vi "piezo.vi"() -> ()   [LabVIEW 2017]
uses:
  C:/Users/Li Lab/Documents/LabVIEW Data/kinesis_test - 3/Thorlabs.MotionControl.Controls.dll
  Thorlabs.MotionControl.Controls.dll
  System.Windows.Forms
  C:/Users/Li Lab/Documents/LabVIEW Data/kinesis_test - 3/Thorlabs.MotionControl.KCube.InertialMotorCLI.dll
  Thorlabs.MotionControl.KCube.InertialMotorCLI.dll
  C:/Users/Li Lab/Documents/LabVIEW Data/kinesis_test - 3/ThorLabs.MotionControl.KCube.DCServoCLI.dll
  ThorLabs.MotionControl.KCube.DCServoCLI.dll
  C:/Program Files/Thorlabs/Scientific Imaging/DCx Camera Support/Develop/DotNet/uc480DotNet.dll
  Program Files/Thorlabs/Scientific Imaging/DCx Camera Support/Develop/DotNet/uc480DotNet.dll
  <vilib>/Utility/inputDevices.llb/mouseAcquire.vi
  <vilib>/Utility/inputDevices.llb/joystickAcquire.vi
  <vilib>/Utility/inputDevices.llb/closeMouse.vi
  <vilib>/Utility/inputDevices.llb/closeJoystick.vi
panel:
  out "blinker and move":bool
  out "in screen?":bool
  in  "ready to use mouse?":bool
  out "Numeric1":dbl
  out "Numeric2":dbl
  out "motor 1":dbl
  out "motor 2":dbl
  out "Moving":bool
  in  "1mm=?pixel":i32
  in  "Motor Display":T1(tab)
  in  "KCubeInertialMotorControl":refnum<k24>(container)
  in  "KCubeDCServoControl-motor 1":refnum<k24>(container)
  in  "KCubeDCServoControl-motor 2":refnum<k24>(container)
  out "error out 9":errorcluster
  out "error out 8":errorcluster
  in  "PictureBox":refnum<k24>(container)
  in  "Init Camera":bool
  in  "Start Live":bool
  in  "Exit Camera":bool
  in  "Stop Live":bool
  in  "Load Parameter":bool
  out "Error Out":errorcluster caption="error"
  out "Bits/Pixel 2":i32=8
  out "Width 2":i32=8
  out "Height 2":i32=8
  out "Serial Number 2":string
  out "Position of z direction":i32
  in  "?":bool
  in  "Input Box":T2(tab)
  in  "a":dbl
  in  "b":dbl
  in  "c":dbl
  in  "d":dbl
  out "upper verti limit":dbl
  out "lower verti limit":dbl
  out "left hori limit":dbl
  out "right hori limit":dbl
  out "Horizontal":i32
  out "Vertical":i32
  out "Scrolling":i32
  out "button 1":bool
  out "button 2":bool
  out "Horizontal right click":i32
  out "Vertical right click":i32
  out "Horizontal left click":i32
  out "Vertical left click":i32
  in  "Pixelclock":i32(slide)=33 min=5 max=43 step=1 scale=5.0..43.0
  in  "Framerate":dbl(slide)=33.21525 min=4.876716604244694 max=13.962044182888818 step=0.013000041138630184 scale=4.876716604244694..13.962044182888818 scale format="%#.3g"
  in  "Exposure":dbl(slide)=33.21525 min=0.06675 max=99.92475 step=0.06675 scale=0.06675..99.92475 scale format="%#.3g"
  in  "Zoom":u16(ring)=1 items=["4X"=4, "2X"=2, "1X"=1]
  in  "Camera ID":i32
  out "Serial Number":string
  out "Height":i32=8
  out "Width":i32=8
  out "Bits/Pixel":i32=8
  in  "SerialNumber KDC101 2":string="27251775"
  in  "SerialNumber KDC101":string="27251750"
  in  "SerialNumber  of KIM101":string="97000019"
  out "Time the program is running (s)":dbl caption="Elapsed Time (s)"
  out "You are Sprinting now":bool
  in  "channel 3":i32(ring)=1 items=["Channel1"=1, "Channel2"=2, "Channel3"=3, "Channel4"=4]
  in  "stop 2":bool
  in  "stop":bool
  in  "Cancel Button":bool
  in  "Move motor control":bool
  in  "step size (mm) 2":dbl
  in  "end pos (mm)":dbl
  out "Move motor indicator":bool
  out "position of motor 2 (mm)":dbl
  out "error out 7":errorcluster
  out "error out 6":errorcluster
  out "error out 4":errorcluster
  out "error out 3":errorcluster
  out "error out 2":errorcluster
  out "error out":errorcluster
  out "error out 5":errorcluster
  out "position of motor 1 (mm)":dbl
  out "direction info 2":T3
  out "axis info 2":T4
  out "button info 2":T5
  # "left is off, right is on"
  # "Li Lab, Camera and Microscope Stage Controller"
  # "1. Right Click on the laser point and left click where you want to move it\n2. Please Exit camera before closing the program, please, please, please!!!!!\n3. Enter the mm to pixel convertion before moving the mouse.\n4. All the input controls can be found on the Input Control Box!\n5. If any Bugs found please contact deyraunak111@gmail.com\n6. A video or photo recording version will come up shortly, until that use the Thorlabs camera.\n7. Set the laser position and the screen before trying to capture the bead with the mouse. Look at the convention and input the \nvalues of a,b,c,d. Then turn the knob to use mouse. Enjoy!"
  # "laser pointer"
  # "Axis convention:"
  # "up is negative down is positiive, right is positive left is negative"
  # "This feature is non functional now for the time being"
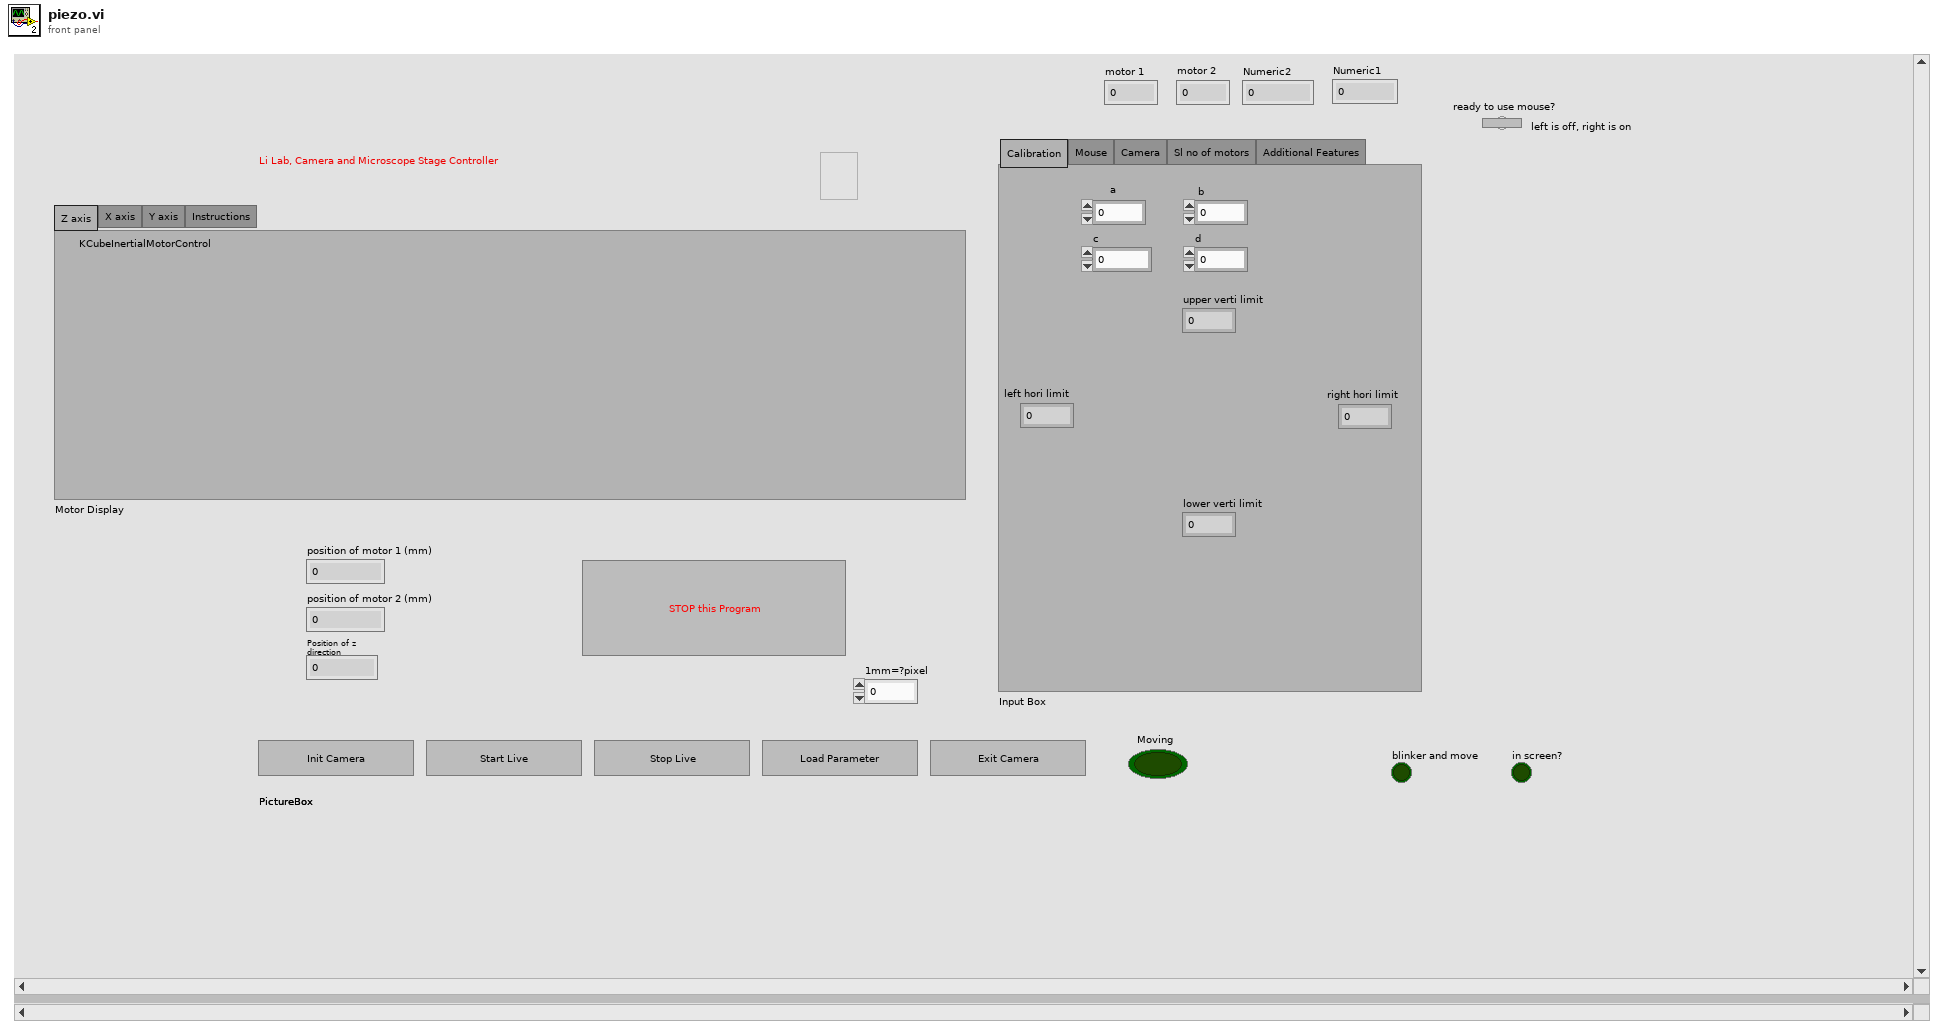
[diagram p1: front panel]
types:
  T1 = enum32{"Z axis", "X axis", "Y axis", "Instructions"}
  T2 = enum32{"Calibration", "Mouse", "Camera", "Sl no of motors", "Additional Features"}
  T3 = cluster{"pov 1":i32, "pov 2":i32, "pov 3":i32, "pov 4":i32}
  T4 = cluster{"X axis":i32, "Y axis":i32, "Z axis":i32, "X axis rotation":i32, "Y axis rotation":i32, "Z axis rotation":i32, "U axis":i32, "V axis":i32}
  T5 = cluster{"button 1":bool, "button 2":bool, "button 3":bool, "button 4":bool, "button 5":bool, "button 6":bool, "button 7":bool, "button 8":bool, "button 9":bool, "button 10":bool, "button 11":bool, "button 12":bool, "button 13":bool, "button 14":bool, "button 15":bool, "button 16":bool, "button 17":bool, "button 18":bool, "button 19":bool, "button 20":bool, "button 21":bool, "button 22":bool, "button 23":bool, "button 24":bool, "button 25":bool, "button 26":bool, "button 27":bool, "button 28":bool, "button 29":bool, "button 30":bool, "button 31":bool, "button 32":bool}
  T6 = enum8{"Enabled", "Disabled", "Disabled and Grayed Out"}
  T7 = cluster{"Horizontal":i32, "Vertical":i32, "Scrolling":i32}
  T8 = cluster{"button 1":bool, "button 2":bool, "button 3":bool, "button 4":bool}
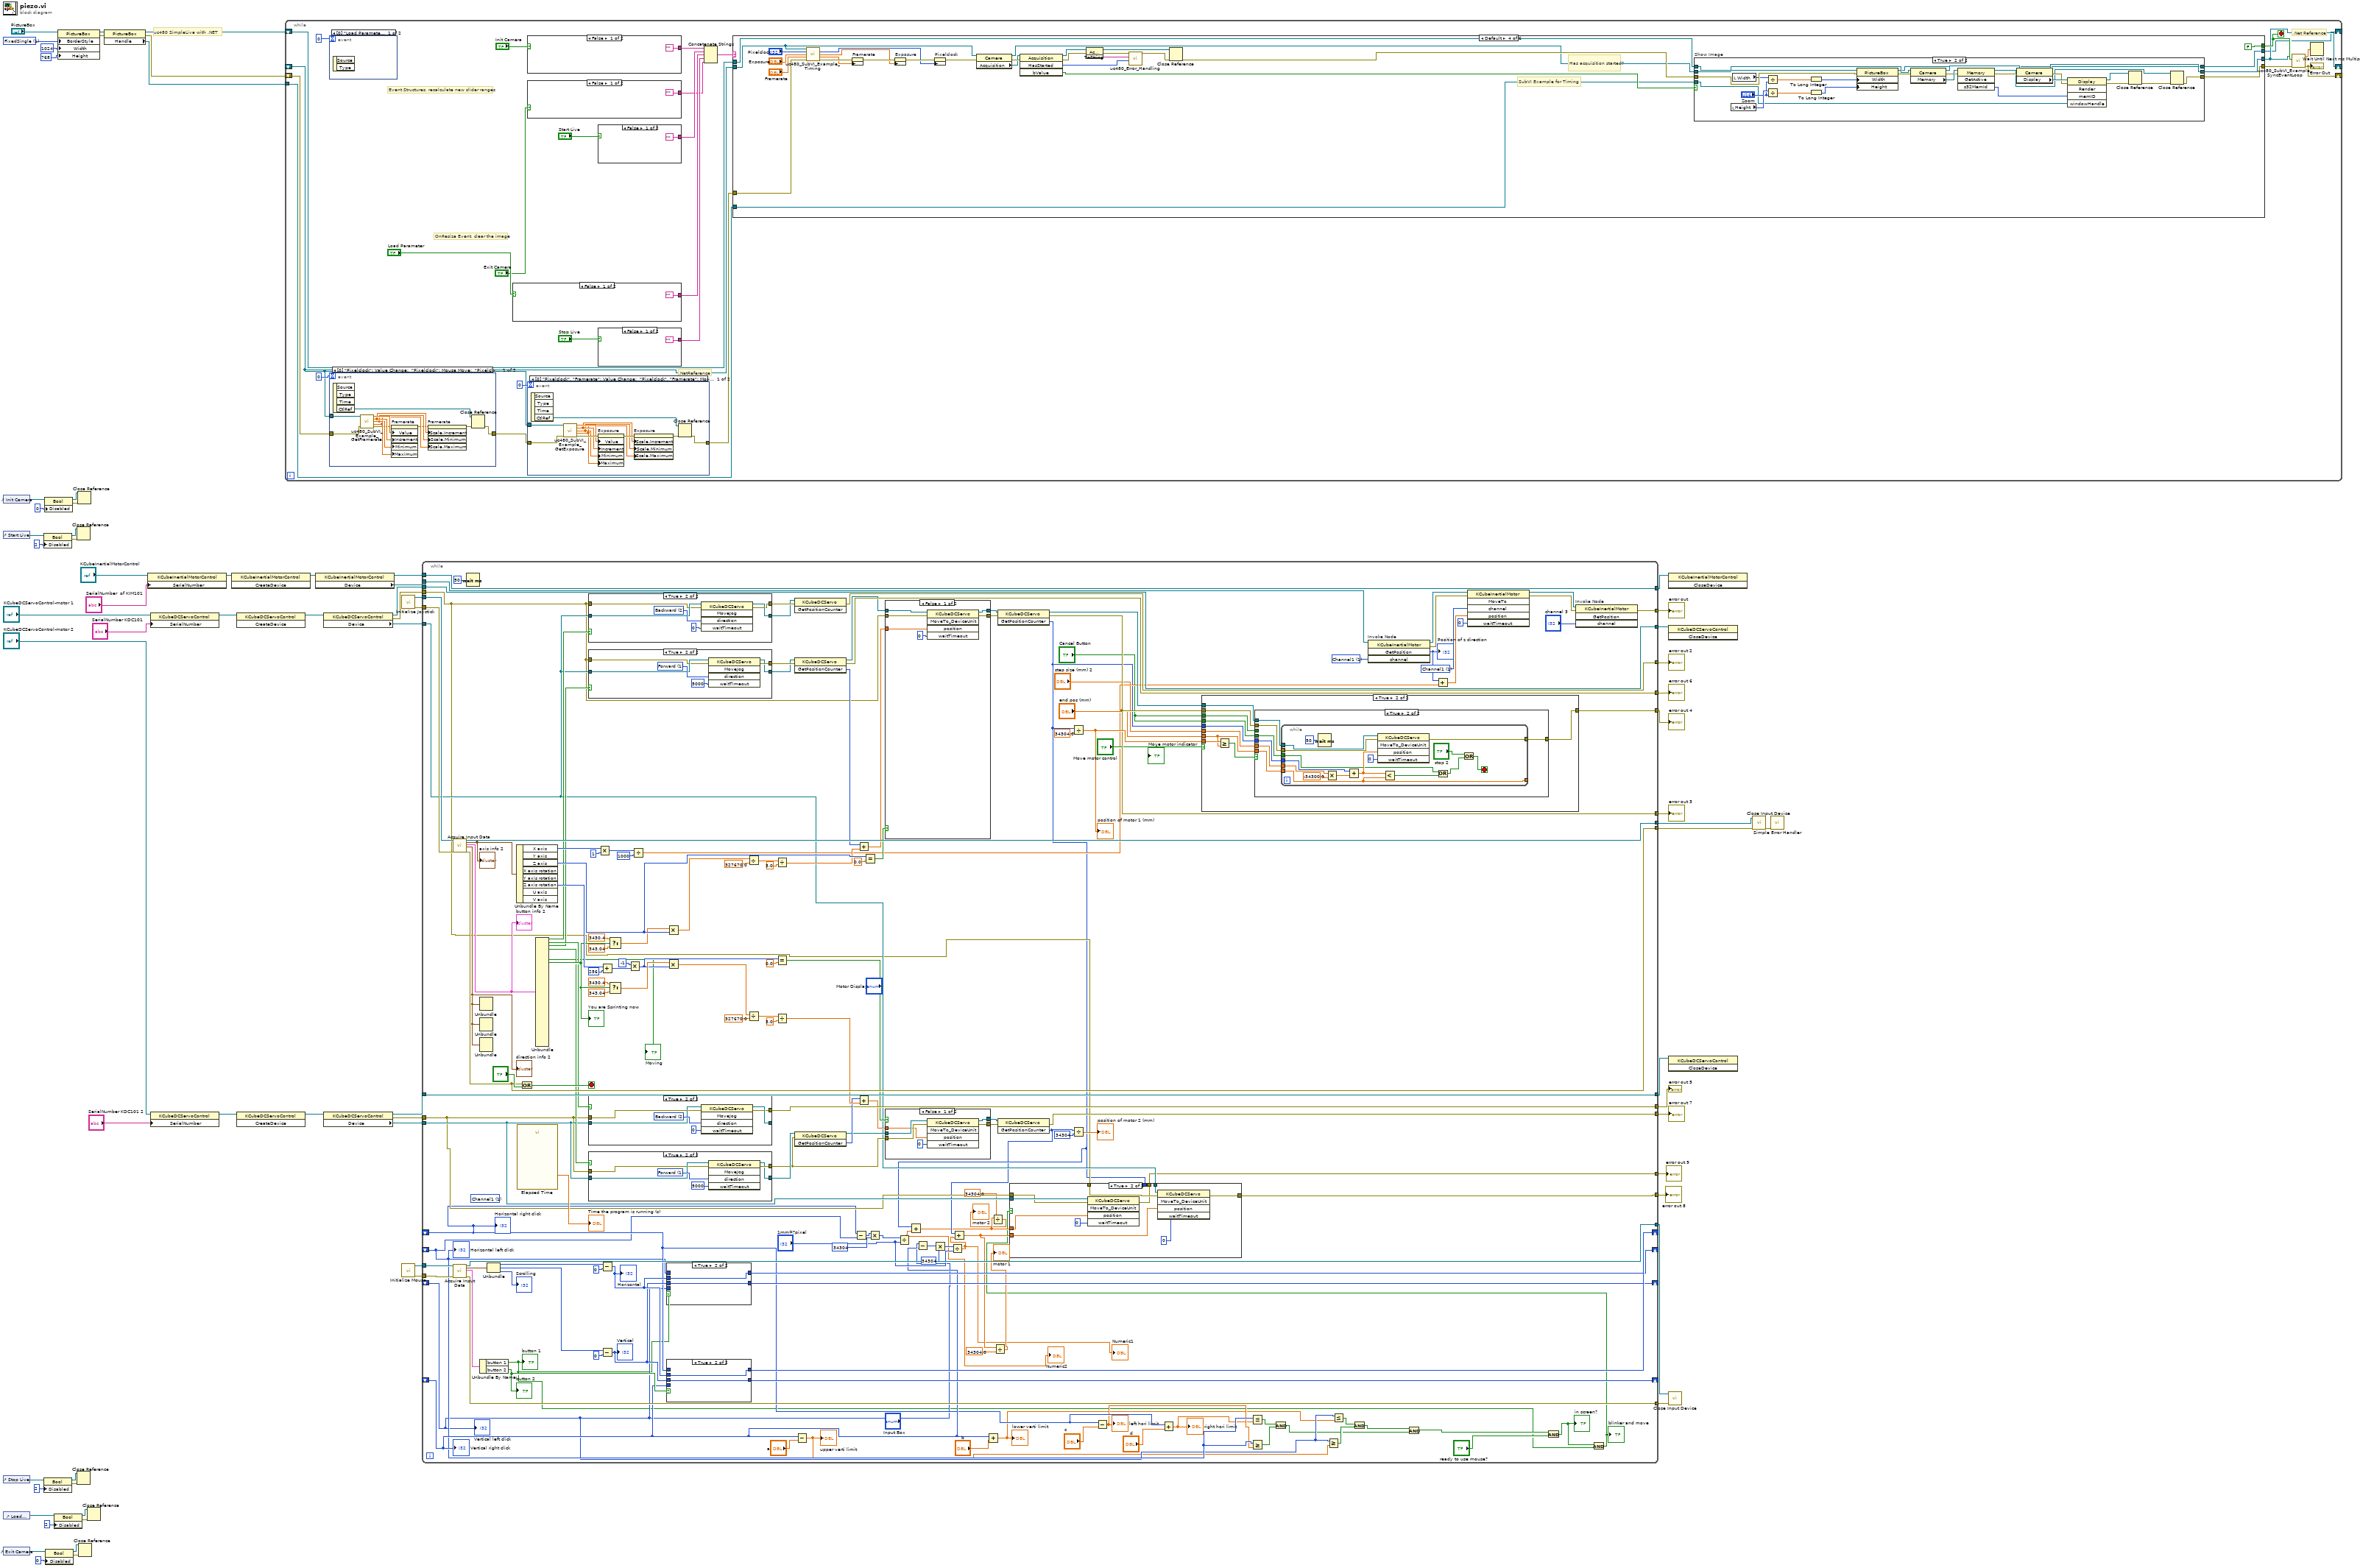
[diagram p0: block diagram]
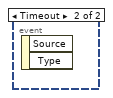
[diagram p2: hidden frame]
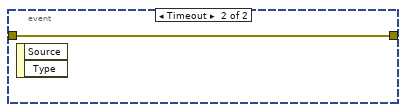
[diagram p3: hidden frame]
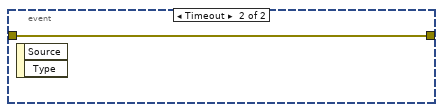
[diagram p4: hidden frame]
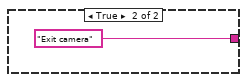
[diagram p5: hidden frame]
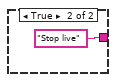
[diagram p6: hidden frame]
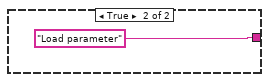
[diagram p7: hidden frame]
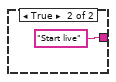
[diagram p8: hidden frame]
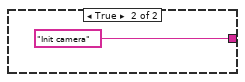
[diagram p9: hidden frame]
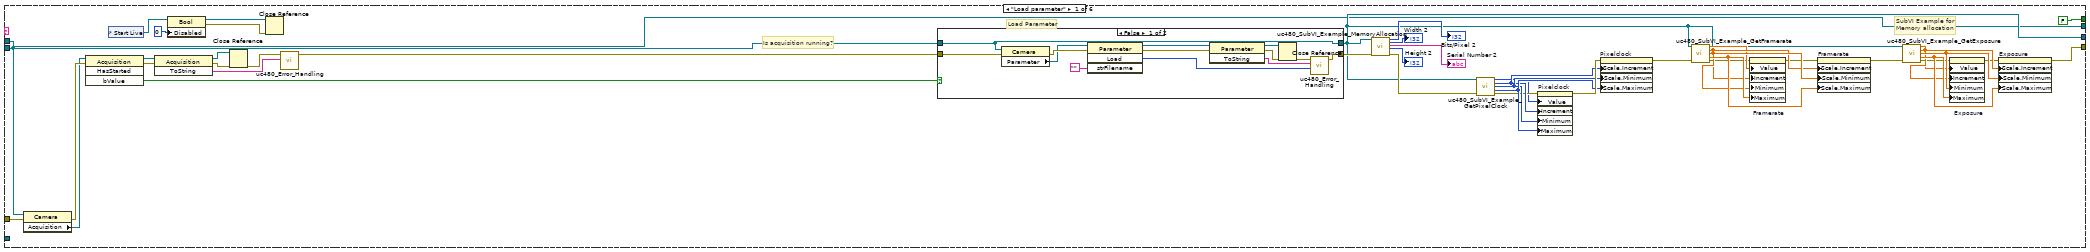
[diagram p10: hidden frame]
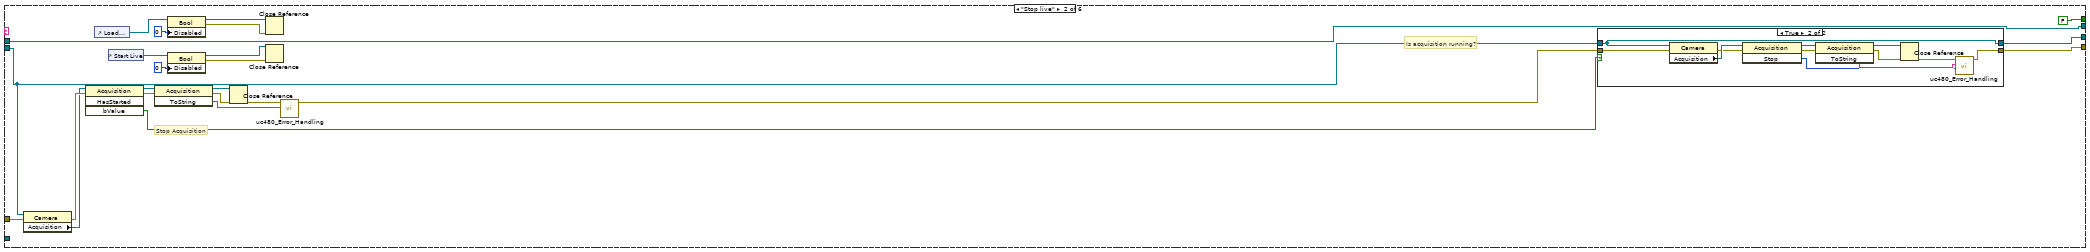
[diagram p12: hidden frame]
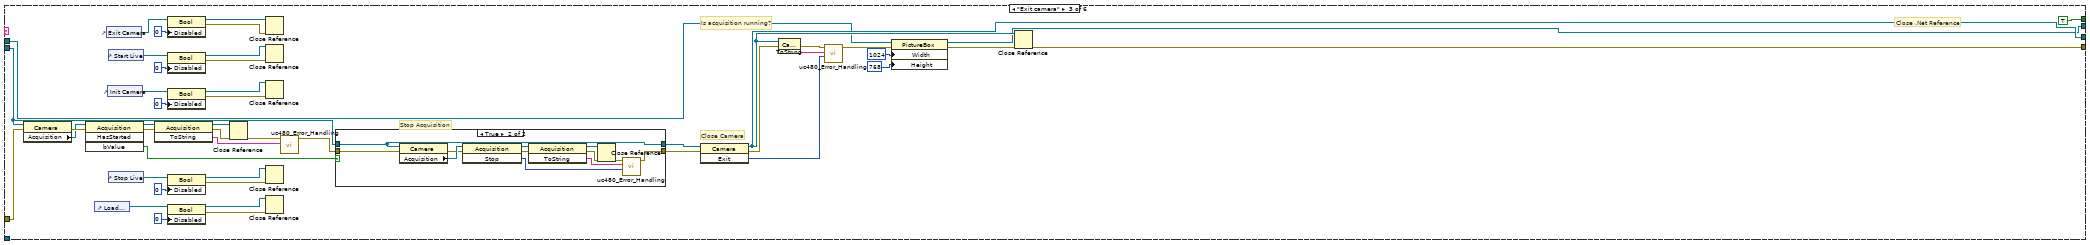
[diagram p14: hidden frame]
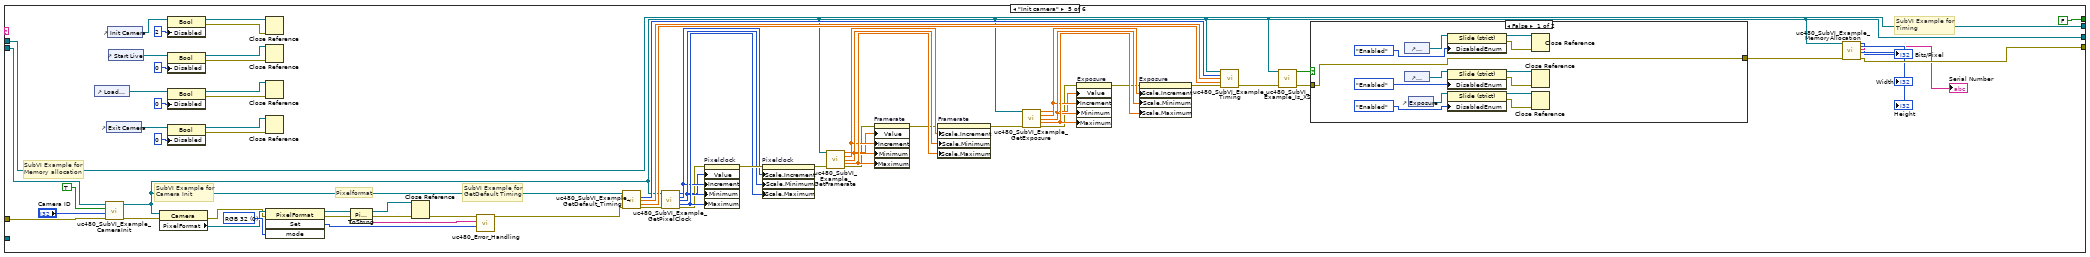
[diagram p17: hidden frame]
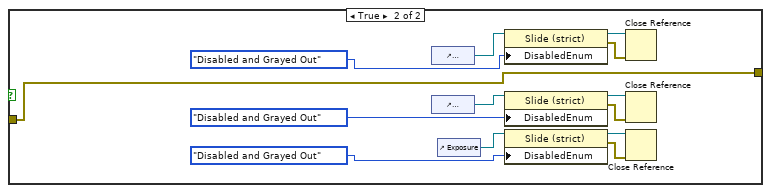
[diagram p18: hidden frame]
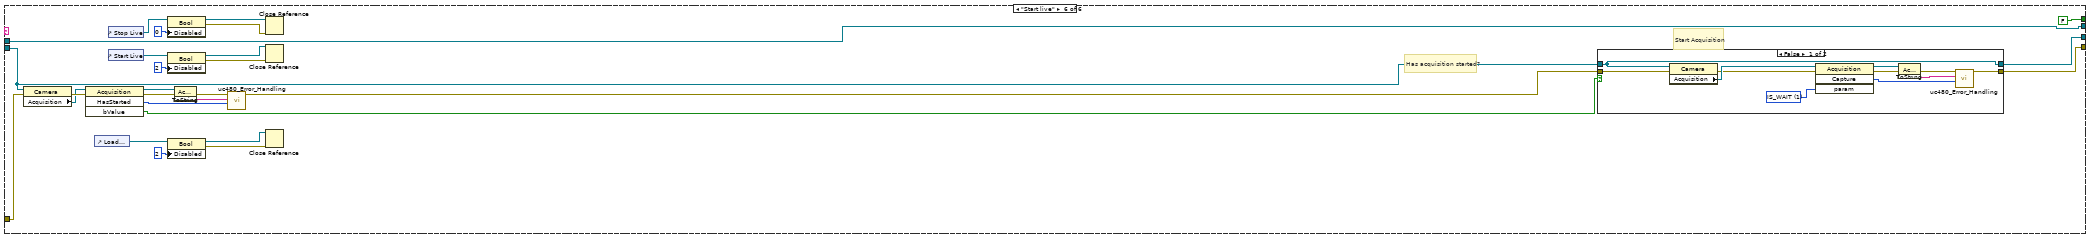
[diagram p19: hidden frame]
diagram:
  w24 = 1 items=["None", "FixedSingle", "Fixed3D"] ("BorderStyle")
  # "uc480 SimpleLive with .NET"
  n1 = control-ref of="Init Camera"() -> (w35:refnum<vi>)
  n2 = control-ref of="Start Live"() -> (w32:refnum<vi>)
  n3 = control-ref of="Stop Live"() -> (w26:refnum<vi>)
  n4 = control-ref of="Load Parameter"() -> (w27:refnum<vi>)
  n5 = control-ref of="Exit Camera"() -> (w28:refnum<vi>)
  n6 = property class="Bool"(reference=w32, "Disabled"=u8 2 ("Deaktiviert")) -> (reference out=w19:refnum<vi>, error out=w18:errorcluster)  [unwired: 1 in]
  n7 = property class="Bool"(reference=w26, "Disabled"=u8 2 ("Deaktiviert")) -> (reference out=w17:refnum<vi>, error out=w16:errorcluster)  [unwired: 1 in]
  n8 = property class="Bool"(reference=w35, "Disabled"=u8 0 ("Deaktiviert")) -> (reference out=w21:refnum<vi>, error out=w20:errorcluster)  [unwired: 1 in]
  n9 = property class="Bool"(reference=w28, "Disabled"=u8 0 ("Deaktiviert")) -> (reference out=w13:refnum<vi>, error out=w12:errorcluster)  [unwired: 1 in]
  n10 = property class="Bool"(reference=w27, "Disabled"=u8 2 ("Deaktiviert")) -> (reference out=w15:refnum<vi>, error out=w14:errorcluster)  [unwired: 1 in]
  n11 = property class="PictureBox"(reference="PictureBox", "BorderStyle"=w24, "Width"=1024, "Height"=768) -> (reference out=w10:refnum<k24>, error out=w11:errorcluster)  [unwired: 1 in]
  n12 = Close Reference(reference=w19, error in (no error)=w18) -> ()  [unwired: 1 out]
  n13 = Close Reference(reference=w17, error in (no error)=w16) -> ()  [unwired: 1 out]
  n14 = Close Reference(reference=w21, error in (no error)=w20) -> ()  [unwired: 1 out]
  n15 = Close Reference(reference=w13, error in (no error)=w12) -> ()  [unwired: 1 out]
  n16 = Close Reference(reference=w15, error in (no error)=w14) -> ()  [unwired: 1 out]
  n17 = property class="PictureBox"(reference=w10, error in=w11) -> (reference out=w9:refnum<k24>, error out=w8:errorcluster, "Handle"=w7:refnum<k24>)
  n18 = property class="KCubeInertialMotorControl"(reference="KCubeInertialMotorControl", "SerialNumber"="SerialNumber  of KIM101") -> (reference out=w68:refnum<k24>)  [unwired: 1 in, 1 out]
  n19 = property class="KCubeDCServoControl"(reference="KCubeDCServoControl-motor 1", "SerialNumber"="SerialNumber KDC101") -> (reference out=w63:refnum<k24>)  [unwired: 1 in, 1 out]
  n20 = property class="KCubeDCServoControl"(reference="KCubeDCServoControl-motor 2", "SerialNumber"="SerialNumber KDC101 2") -> (reference out=w58:refnum<k24>)  [unwired: 1 in, 1 out]
  n21 = invoke class="KCubeInertialMotorControl" method="CreateDevice"(reference=w68) -> (reference out=w67:refnum<k24>)  [unwired: 2 in, 2 out]
  n22 = invoke class="KCubeDCServoControl" method="CreateDevice"(reference=w63) -> (reference out=w64:refnum<k24>)  [unwired: 2 in, 2 out]
  n23 = invoke class="KCubeDCServoControl" method="CreateDevice"(reference=w58) -> (reference out=w57:refnum<k24>)  [unwired: 2 in, 2 out]
  n24 = while {
    shift-right: [w75] -> _
    shift-left: w8 -> [w81]
    shift-right: [w78] -> _
    shift-left: _ -> [w71]
    shift-right: [w73] -> _
    shift-left: w9 -> [w74]
    tunnel: w7 -> [w72]
    stop <- w79 stop-if-true
    # "OnResize Event, clear the image"
    # "Event Structures, recalculate new slider ranges"
    # ".NetReference"
    # ".Net Reference"
    n25 = event shown="[0] \"Load Parameter\", \"Start Live\": Mouse Down" {
      selector: _ -> [_ _]
      dyn-events: _ -> [_ _]
      timeout: 0 -> [_ _]
      event "Load Parameter", "Start Live": Mouse Down {
        n26 = event-data() -> ()  [unwired: 1 in, 2 out]
      }
      event Timeout {
        n27 = event-data() -> ()  [unwired: 1 in, 2 out]
      }
    }
    n28 = event shown="[0] \"Pixelclock\": Value Change;  \"Pixelclock\": Mouse Move;  \"Pixelclock\": Key Down;  \"Pixelclock\": Mouse Up" {
      selector: _ -> [_ _]
      dyn-events: _ -> [_ _]
      timeout: 0 -> [_ _]
      tunnel: [w97 w108] -> w82
      tunnel: w81 -> [w107 w108]
      tunnel: w71 -> [w106 _]
      event "Pixelclock": Value Change; "Pixelclock": Mouse Move; "Pixelclock": Key Down; "Pixelclock": Mouse Up {
        n29 = event-data() -> ("CtlRef"=w99:refnum<vi>)  [unwired: 1 in, 3 out]
        n30 = call "uc480_SubVI_Example_GetFramerate.vi"(".NET (Reference)"=w106, "Error In"=w107) -> ("Framerate"=w105:dbl, "Inc"=w104:dbl, "Min"=w102:dbl, "Max"=w103:dbl, "error out"=w101:errorcluster)  [unwired: 9 in]
        n31 = property on="Framerate" class="Slide (strict)"(error in=w101, "Value"=w105, "Increment"=w104, "Minimum"=w102, "Maximum"=w103) -> (error out=w100:errorcluster)  [unwired: 1 in, 1 out]
        n32 = property on="Framerate" class="Slide (strict)"(error in=w100, "Scale.Increment"=w104, "Scale.Minimum"=w102, "Scale.Maximum"=w103) -> (error out=w98:errorcluster)  [unwired: 1 in, 1 out]
        n33 = Close Reference(reference=w99, error in (no error)=w98) -> (error out=w97:errorcluster)
      }
      event Timeout {
        n34 = event-data() -> ()  [unwired: 1 in, 2 out]
      }
    }
    n35 = case shown="False" "Load Parameter" {
      tunnel: ["" "Load parameter"] -> w90
      frame False {
      }
      frame True {
      }
    }
    n36 = case shown="False" "Init Camera" {
      tunnel: ["" "Init camera"] -> w94
      frame False {
      }
      frame True {
      }
    }
    n37 = case shown="False" "Exit Camera" {
      tunnel: ["" "Exit camera"] -> w86
      frame False {
      }
      frame True {
      }
    }
    n38 = event shown="[0] \"Pixelclock\", \"Framerate\": Value Change;  \"Pixelclock\", \"Framerate\": Mouse Move;  \"Pixelclock\", \"Framerate\": Key Down;  \"Pixelclock\", \"Framerate\": Mouse Up" {
      selector: _ -> [_ _]
      dyn-events: _ -> [_ _]
      timeout: 0 -> [_ _]
      tunnel: w82 -> [w119 w120]
      tunnel: [w109 w120] -> w84
      tunnel: w71 -> [w118 _]
      event "Pixelclock", "Framerate": Value Change; "Pixelclock", "Framerate": Mouse Move; "Pixelclock", "Framerate": Key Down; "Pixelclock", "Framerate": Mouse Up {
        n39 = event-data() -> ("CtlRef"=w111:refnum<vi>)  [unwired: 1 in, 3 out]
        n40 = call "uc480_SubVI_Example_GetExposure.vi"(".NET (Reference)"=w118, "Error In"=w119) -> ("Exposure"=w115:dbl, "Inc"=w114:dbl, "Min"=w113:dbl, "Max"=w112:dbl, "Error out"=w116:errorcluster)  [unwired: 9 in]
        n41 = property on="Exposure" class="Slide (strict)"(error in=w116, "Value"=w115, "Increment"=w114, "Minimum"=w113, "Maximum"=w112) -> (error out=w117:errorcluster)  [unwired: 1 in, 1 out]
        n42 = property on="Exposure" class="Slide (strict)"(error in=w117, "Scale.Increment"=w114, "Scale.Minimum"=w113, "Scale.Maximum"=w112) -> (error out=w110:errorcluster)  [unwired: 1 in, 1 out]
        n43 = Close Reference(reference=w111, error in (no error)=w110) -> (error out=w109:errorcluster)
      }
      event Timeout {
        n44 = event-data() -> ()  [unwired: 1 in, 2 out]
      }
    }
    n45 = case shown="False" "Start Live" {
      tunnel: ["" "Start live"] -> w93
      frame False {
      }
      frame True {
      }
    }
    n46 = case shown="False" "Stop Live" {
      tunnel: ["" "Stop live"] -> w89
      frame False {
      }
      frame True {
      }
    }
    n47 = Concatenate Strings(w94, w93, w90, w89, w86) -> (w92:string)
    n48 = case shown="Default" w92 {
      tunnel: w71 -> [w167 w207 w261 w303 w410 w461]
      tunnel: w84 -> [w170 w208 w262 w313 w409 w462]
      tunnel: [w137 w206 w270 w312 w366 w460] -> w78
      tunnel: [w138 w205 w271 w311 w405 w458] -> w77
      tunnel: [FALSE FALSE TRUE FALSE FALSE FALSE] -> w79
      tunnel: w74 -> [w136 w199 w241 w295 w361 w451]
      tunnel: [w136 w199 w240 w294 w361 w451] -> w73
      tunnel: w72 -> [_ _ _ w291 _ _]
      frame "Load parameter" {
        # "SubVI Example for \nMemory allocation"
        # "Is acquisition running?"
        # "Load Parameter"
        n49 = property class="Camera"(reference=w167, error in=w170) -> (error out=w175:errorcluster, "Acquisition"=w174:refnum<k24>)  [unwired: 1 out]
        n50 = invoke class="Acquisition" method="HasStarted"(reference=w174, error in=w175) -> (reference out=w171:refnum<k24>, error out=w173:errorcluster, "bValue"=w169:bool)  [unwired: 2 in, 1 out]
        n51 = control-ref of="Start Live"() -> (w161:refnum<vi>)
        n52 = invoke class="Acquisition" method="ToString"(reference=w171, error in=w173) -> (reference out=w133:refnum<k24>, error out=w132:errorcluster, "ToString"=w172:string)  [unwired: 1 in]
        n53 = property class="Bool"(reference=w161, "Disabled"=u8 0 ("Deaktiviert")) -> (reference out=w135:refnum<vi>, error out=w134:errorcluster)  [unwired: 1 in]
        n54 = Close Reference(reference=w133, error in (no error)=w132) -> (error out=w131:errorcluster)
        n55 = Close Reference(reference=w135, error in (no error)=w134) -> ()  [unwired: 1 out]
        n56 = call "uc480_Error_Handling.vi"("Error String"=w172, "Error In"=w131) -> ("Error Out"=w168:errorcluster)  [unwired: 9 in]
        n57 = case shown="False" w169 {
          tunnel: w168 -> [w183 w190]
          tunnel: w167 -> [w181 w191]
          tunnel: [w182 w190] -> w162
          tunnel: [w181 w191] -> w137
          frame False {
            n58 = property class="Camera"(reference=w181, error in=w183) -> (error out=w185:errorcluster, "Parameter"=w184:refnum<k24>)  [unwired: 1 out]
            n59 = invoke class="Parameter" method="Load"(reference=w184, error in=w185, "strFilename"="") -> (reference out=w187:refnum<k24>, error out=w188:errorcluster, "Load"=w180:i32)  [unwired: 1 in, 1 out]
            n60 = invoke class="Parameter" method="ToString"(reference=w187, error in=w188) -> (reference out=w177:refnum<k24>, error out=w179:errorcluster, "ToString"=w189:string)  [unwired: 1 in]
            n61 = Close Reference(reference=w177, error in (no error)=w179) -> (error out=w178:errorcluster)
            n62 = call "uc480_Error_Handling.vi"("Error Code"=w180, "Error String"=w189, "Error In"=w178) -> ("Error Out"=w182:errorcluster)  [unwired: 8 in]
          }
          frame True {
          }
        }
        n63 = call "uc480_SubVI_Example_MemoryAllocation.vi"(".NET (Reference)"=w137, "Error In"=w162) -> ("Bits/Pixel 2"=→"Bits/Pixel 2":i32, "Width"=→"Width 2":i32, "Serial Number"=→"Serial Number 2":string, "Height"=→"Height 2":i32, "Error Out"=w139:errorcluster)  [unwired: 13 in]
        n64 = call "uc480_SubVI_Example_GetPixelClock.vi"(".NET (Reference)"=w137, "Error In"=w139) -> ("Pixel Clock"=w140:i32, "Inc"=w142:i32, "Min"=w143:i32, "Max"=w144:i32, "error out"=w141:errorcluster)  [unwired: 9 in]
        n65 = property on="Pixelclock" class="Slide (strict)"(error in=w141, "Value"=w140, "Increment"=w142, "Minimum"=w143, "Maximum"=w144) -> (error out=w145:errorcluster)  [unwired: 1 in, 1 out]
        n66 = property on="Pixelclock" class="Slide (strict)"(error in=w145, "Scale.Increment"=w142, "Scale.Minimum"=w143, "Scale.Maximum"=w144) -> (error out=w146:errorcluster)  [unwired: 1 in, 1 out]
        n67 = call "uc480_SubVI_Example_GetFramerate.vi"(".NET (Reference)"=w137, "Error In"=w146) -> ("Framerate"=w149:dbl, "Inc"=w150:dbl, "Min"=w151:dbl, "Max"=w152:dbl, "error out"=w148:errorcluster)  [unwired: 9 in]
        n68 = property on="Framerate" class="Slide (strict)"(error in=w148, "Value"=w149, "Increment"=w150, "Minimum"=w151, "Maximum"=w152) -> (error out=w147:errorcluster)  [unwired: 1 in, 1 out]
        n69 = property on="Framerate" class="Slide (strict)"(error in=w147, "Scale.Increment"=w150, "Scale.Minimum"=w151, "Scale.Maximum"=w152) -> (error out=w153:errorcluster)  [unwired: 1 in, 1 out]
        n70 = call "uc480_SubVI_Example_GetExposure.vi"(".NET (Reference)"=w137, "Error In"=w153) -> ("Exposure"=w156:dbl, "Inc"=w157:dbl, "Min"=w158:dbl, "Max"=w159:dbl, "Error out"=w154:errorcluster)  [unwired: 9 in]
        n71 = property on="Exposure" class="Slide (strict)"(error in=w154, "Value"=w156, "Increment"=w157, "Minimum"=w158, "Maximum"=w159) -> (error out=w155:errorcluster)  [unwired: 1 in, 1 out]
        n72 = property on="Exposure" class="Slide (strict)"(error in=w155, "Scale.Increment"=w157, "Scale.Minimum"=w158, "Scale.Maximum"=w159) -> (error out=w138:errorcluster)  [unwired: 1 in, 1 out]
      }
      frame "Stop live" {
        # "Is acquisition running?"
        # "Stop Acquisition"
        n73 = property class="Camera"(reference=w207, error in=w208) -> (error out=w215:errorcluster, "Acquisition"=w214:refnum<k24>)  [unwired: 1 out]
        n74 = invoke class="Acquisition" method="HasStarted"(reference=w214, error in=w215) -> (reference out=w209:refnum<k24>, error out=w211:errorcluster, "bValue"=w213:bool)  [unwired: 2 in, 1 out]
        n75 = control-ref of="Load Parameter"() -> (w203:refnum<vi>)
        n76 = control-ref of="Start Live"() -> (w200:refnum<vi>)
        n77 = invoke class="Acquisition" method="ToString"(reference=w209, error in=w211) -> (reference out=w192:refnum<k24>, error out=w194:errorcluster, "ToString"=w210:string)  [unwired: 1 in]
        n78 = property class="Bool"(reference=w203, "Disabled"=u8 0 ("Deaktiviert")) -> (reference out=w198:refnum<vi>, error out=w197:errorcluster)  [unwired: 1 in]
        n79 = property class="Bool"(reference=w200, "Disabled"=u8 0 ("Deaktiviert")) -> (reference out=w196:refnum<vi>, error out=w195:errorcluster)  [unwired: 1 in]
        n80 = Close Reference(reference=w192, error in (no error)=w194) -> (error out=w193:errorcluster)
        n81 = Close Reference(reference=w198, error in (no error)=w197) -> ()  [unwired: 1 out]
        n82 = Close Reference(reference=w196, error in (no error)=w195) -> ()  [unwired: 1 out]
        n83 = call "uc480_Error_Handling.vi"("Error String"=w210, "Error In"=w193) -> ("Error Out"=w212:errorcluster)  [unwired: 9 in]
        n84 = case shown="True" w213 {
          tunnel: [w217 w228] -> w205
          tunnel: w212 -> [w217 w229]
          tunnel: w207 -> [w216 w221]
          tunnel: [w216 w221] -> w206
          frame False {
          }
          frame True {
            n85 = property class="Camera"(reference=w221, error in=w229) -> (error out=w225:errorcluster, "Acquisition"=w226:refnum<k24>)  [unwired: 1 out]
            n86 = invoke class="Acquisition" method="Stop"(reference=w226, error in=w225) -> (reference out=w223:refnum<k24>, error out=w224:errorcluster, "Stop"=w222:i32)  [unwired: 1 in]
            n87 = invoke class="Acquisition" method="ToString"(reference=w223, error in=w224) -> (reference out=w218:refnum<k24>, error out=w220:errorcluster, "ToString"=w227:string)  [unwired: 1 in]
            n88 = Close Reference(reference=w218, error in (no error)=w220) -> (error out=w219:errorcluster)
            n89 = call "uc480_Error_Handling.vi"("Error Code"=w222, "Error String"=w227, "Error In"=w219) -> ("Error Out"=w228:errorcluster)  [unwired: 8 in]
          }
        }
      }
      frame "Exit camera" {
        # "Close .Net Reference"
        # "Is acquisition running?"
        # "Stop Acquisition"
        # "Close Camera"
        n90 = property class="Camera"(reference=w261, error in=w262) -> (error out=w269:errorcluster, "Acquisition"=w268:refnum<k24>)  [unwired: 1 out]
        n91 = invoke class="Acquisition" method="HasStarted"(reference=w268, error in=w269) -> (reference out=w263:refnum<k24>, error out=w265:errorcluster, "bValue"=w267:bool)  [unwired: 2 in, 1 out]
        n92 = control-ref of="Load Parameter"() -> (w251:refnum<vi>)
        n93 = control-ref of="Exit Camera"() -> (w249:refnum<vi>)
        n94 = control-ref of="Init Camera"() -> (w253:refnum<vi>)
        n95 = control-ref of="Start Live"() -> (w252:refnum<vi>)
        n96 = control-ref of="Stop Live"() -> (w250:refnum<vi>)
        n97 = invoke class="Acquisition" method="ToString"(reference=w263, error in=w265) -> (reference out=w246:refnum<k24>, error out=w248:errorcluster, "ToString"=w264:string)  [unwired: 1 in]
        n98 = property class="Bool"(reference=w249, "Disabled"=u8 0 ("Deaktiviert")) -> (reference out=w239:refnum<vi>, error out=w238:errorcluster)  [unwired: 1 in]
        n99 = property class="Bool"(reference=w252, "Disabled"=u8 0 ("Deaktiviert")) -> (reference out=w233:refnum<vi>, error out=w232:errorcluster)  [unwired: 1 in]
        n100 = property class="Bool"(reference=w253, "Disabled"=u8 0 ("Deaktiviert")) -> (reference out=w231:refnum<vi>, error out=w230:errorcluster)  [unwired: 1 in]
        n101 = property class="Bool"(reference=w250, "Disabled"=u8 0 ("Deaktiviert")) -> (reference out=w237:refnum<vi>, error out=w236:errorcluster)  [unwired: 1 in]
        n102 = property class="Bool"(reference=w251, "Disabled"=u8 0 ("Deaktiviert")) -> (reference out=w235:refnum<vi>, error out=w234:errorcluster)  [unwired: 1 in]
        n103 = Close Reference ("Close Referenz")(reference=w246, error in (no error)=w248) -> (error out=w247:errorcluster)
        n104 = Close Reference(reference=w239, error in (no error)=w238) -> ()  [unwired: 1 out]
        n105 = Close Reference(reference=w233, error in (no error)=w232) -> ()  [unwired: 1 out]
        n106 = Close Reference(reference=w231, error in (no error)=w230) -> ()  [unwired: 1 out]
        n107 = Close Reference(reference=w237, error in (no error)=w236) -> ()  [unwired: 1 out]
        n108 = Close Reference(reference=w235, error in (no error)=w234) -> ()  [unwired: 1 out]
        n109 = call "uc480_Error_Handling.vi"("Error String"=w264, "Error In"=w247) -> ("Error Out"=w266:errorcluster)  [unwired: 9 in]
        n110 = case shown="True" w267 {
          tunnel: [w278 w289] -> w259
          tunnel: w266 -> [w278 w290]
          tunnel: w261 -> [w277 w282]
          tunnel: [w277 w282] -> w260
          frame False {
          }
          frame True {
            n111 = property class="Camera"(reference=w282, error in=w290) -> (error out=w286:errorcluster, "Acquisition"=w287:refnum<k24>)  [unwired: 1 out]
            n112 = invoke class="Acquisition" method="Stop"(reference=w287, error in=w286) -> (reference out=w284:refnum<k24>, error out=w285:errorcluster, "Stop"=w283:i32)  [unwired: 1 in]
            n113 = invoke class="Acquisition" method="ToString"(reference=w284, error in=w285) -> (reference out=w279:refnum<k24>, error out=w281:errorcluster, "ToString"=w288:string)  [unwired: 1 in]
            n114 = Close Reference ("Close Referenz")(reference=w279, error in (no error)=w281) -> (error out=w280:errorcluster)
            n115 = call "uc480_Error_Handling.vi"("Error Code"=w283, "Error String"=w288, "Error In"=w280) -> ("Error Out"=w289:errorcluster)  [unwired: 8 in]
          }
        }
        n116 = invoke class="Camera" method="Exit"(reference=w260, error in=w259) -> (reference out=w270:refnum<k24>, error out=w273:errorcluster, "Exit"=w272:i32)  [unwired: 1 in]
        n117 = invoke class="Camera" method="ToString"(reference=w270, error in=w273) -> (error out=w274:errorcluster, "ToString"=w275:string)  [unwired: 1 in, 1 out]
        n118 = call "uc480_Error_Handling.vi"("Error Code"=w272, "Error String"=w275, "Error In"=w274) -> ("Error Out"=w245:errorcluster)  [unwired: 8 in]
        n119 = property class="PictureBox"(reference=w241, error in=w245, "Width"=1024, "Height"=768) -> (reference out=w240:refnum<k24>, error out=w244:errorcluster)
        n120 = Close Reference ("Close Referenz")(reference=w270, error in (no error)=w244) -> (error out=w271:errorcluster)
      }
      frame Default {
        # "SubVI Example for Timing"
        # "Has acquisition started?"
        n121 = call "uc480_SubVI_Example_Timing.vi"(".NET (Reference)"=w303, "Pixelclock"="Pixelclock", "Exposure time"="Exposure", "Framerate"="Framerate", "Error In"=w313) -> ("Pixelclock"=w306:i32, "Exposure time"=w305:dbl, "Framerate"=w304:dbl, "Error Out"=w310:errorcluster)  [unwired: 7 in]
        n122 = property on="Framerate" class="Schieber (strikt)"(error in=w310, "Scale.RngStart"=w304) -> (error out=w309:errorcluster)  [unwired: 1 in, 1 out]
        n123 = property on="Exposure" class="Schieber (strikt)"(error in=w309, "Scale.RngStart"=w305) -> (error out=w308:errorcluster)  [unwired: 1 in, 1 out]
        n124 = property on="Pixelclock" class="Schieber (strikt)"(error in=w308, "Scale.RngStart"=w306) -> (error out=w307:errorcluster)  [unwired: 1 in, 1 out]
        n125 = property class="Camera"(reference=w303, error in=w307) -> (reference out=w296:refnum<k24>, error out=w319:errorcluster, "Acquisition"=w318:refnum<k24>)
        n126 = invoke class="Acquisition" method="HasStarted"(reference=w318, error in=w319) -> (reference out=w293:refnum<k24>, error out=w315:errorcluster, "HasStarted"=w314:i32, "bValue"=w292:bool)  [unwired: 2 in]
        n127 = invoke class="Acquisition" method="ToString"(reference=w293, error in=w315) -> (reference out=w297:refnum<k24>, error out=w317:errorcluster, "ToString"=w316:string)  [unwired: 1 in]
        n128 = call "uc480_Error_Handling.vi"("Error Code"=w314, "Error String"=w316, "Error In"=w317) -> ("Error Out"=w299:errorcluster)  [unwired: 8 in]
        n129 = Close Reference(reference=w297, error in (no error)=w299) -> (error out=w298:errorcluster)
        n130 = case "Show Image" shown="True" w292 {
          tunnel: [w323 w329] -> w311
          tunnel: w298 -> [w323 w340]
          tunnel: w296 -> [w322 w339]
          tunnel: [w322 w344] -> w312
          tunnel: w295 -> [w321 w341]
          tunnel: [w321 w325] -> w294
          tunnel: w291 -> [_ w324]
          frame False {
          }
          frame True {
            n131 = local read "Height"() -> (w337:i32)
            n132 = local read "Width"() -> (w333:i32)
            n133 = Divide(x=w333, y="Zoom") -> (x/y=w335:dbl)
            n134 = Divide(x=w337, y="Zoom") -> (x/y=w338:dbl)
            n135 = To Long Integer(number=w335) -> (32bit integer=w334:i32)
            n136 = To Long Integer(number=w338) -> (32bit integer=w336:i32)
            n137 = property class="PictureBox"(reference=w341, error in=w340, "Width"=w334, "Height"=w336) -> (reference out=w325:refnum<k24>, error out=w326:errorcluster)
            n138 = property class="Camera"(reference=w339, error in=w326) -> (reference out=w345:refnum<k24>, error out=w348:errorcluster, "Memory"=w349:refnum<k24>)
            n139 = invoke class="Memory" method="GetActive"(reference=w349, error in=w348) -> (reference out=w327:refnum<k24>, error out=w328:errorcluster, "s32MemId"=w343:i32)  [unwired: 2 in, 1 out]
            n140 = property class="Camera"(reference=w345, error in=w328) -> (reference out=w344:refnum<k24>, error out=w342:errorcluster, "Display"=w347:refnum<k24>)
            n141 = invoke class="Display" method="Render"(reference=w347, error in=w342, "memID"=w343, "windowHandle"=w324) -> (reference out=w346:refnum<k24>, error out=w331:errorcluster)  [unwired: 1 in, 3 out]
            n142 = Close Reference(reference=w346, error in (no error)=w331) -> (error out=w330:errorcluster)
            n143 = Close Reference(reference=w327, error in (no error)=w330) -> (error out=w329:errorcluster)
          }
        }
      }
      frame "Init camera" {
        w418 = 0 items=["RGB 32"=0, "RGB 24"=1, "Y8 Monochrom"=6] ("Mode")
        # "SubVI Example for \nGetDefault Timing"
        # "SubVI Example for \nMemory allocation"
        # "SubVI Example for \nTiming"
        # "SubVI Example for \nCamera Init"
        # "Pixelformat"
        n144 = control-ref of="Load Parameter"() -> (w369:refnum<vi>)
        n145 = call "uc480_SubVI_Example_CameraInit.vi"("Error In"=w409, "Camera ID"="Camera ID", "Init Camera Flag"=TRUE, ".NET (Reference)"=w410) -> ("Error Out"=w415:errorcluster, ".NET (Reference)"=w366:refnum<k24>)  [unwired: 6 in]
        n146 = control-ref of="Exit Camera"() -> (w367:refnum<vi>)
        n147 = control-ref of="Init Camera"() -> (w373:refnum<vi>)
        n148 = control-ref of="Start Live"() -> (w371:refnum<vi>)
        n149 = property on="Property Node" class="Camera"(reference=w366, error in=w415) -> (error out=w416:errorcluster, "PixelFormat"=w417:refnum<k24>)  [unwired: 1 out]
        n150 = property class="Bool"(reference=w373, "Disabled"=u8 2 ("Deaktiviert")) -> (reference out=w360:refnum<vi>, error out=w359:errorcluster)  [unwired: 1 in]
        n151 = property class="Bool"(reference=w371, "Disabled"=u8 0 ("Deaktiviert")) -> (reference out=w358:refnum<vi>, error out=w357:errorcluster)  [unwired: 1 in]
        n152 = property class="Bool"(reference=w369, "Disabled"=u8 0 ("Deaktiviert")) -> (reference out=w356:refnum<vi>, error out=w355:errorcluster)  [unwired: 1 in]
        n153 = property class="Bool"(reference=w367, "Disabled"=u8 0 ("Deaktiviert")) -> (reference out=w354:refnum<vi>, error out=w353:errorcluster)  [unwired: 1 in]
        n154 = Close Reference(reference=w360, error in (no error)=w359) -> ()  [unwired: 1 out]
        n155 = Close Reference(reference=w358, error in (no error)=w357) -> ()  [unwired: 1 out]
        n156 = Close Reference(reference=w356, error in (no error)=w355) -> ()  [unwired: 1 out]
        n157 = Close Reference(reference=w354, error in (no error)=w353) -> ()  [unwired: 1 out]
        n158 = invoke class="PixelFormat" method="Set"(reference=w417, error in=w416, "mode"=w418) -> (reference out=w413:refnum<k24>, error out=w406:errorcluster, "Set"=w412:i32)  [unwired: 1 in, 1 out]
        n159 = invoke class="PixelFormat" method="ToString"(reference=w413, error in=w406) -> (reference out=w350:refnum<k24>, error out=w352:errorcluster, "ToString"=w414:string)  [unwired: 1 in]
        n160 = Close Reference(reference=w350, error in (no error)=w352) -> (error out=w351:errorcluster)
        n161 = call "uc480_Error_Handling.vi"("Error Code"=w412, "Error String"=w414, "Error In"=w351) -> ("Error Out"=w380:errorcluster)  [unwired: 8 in]
        n162 = call "uc480_SubVI_Example_GetDefault_Timing.vi"(".NET (Reference)"=w366, "Error In"=w380) -> ("Pixelclock"=w379:i32, "Exposure time"=w378:dbl, "Framerate"=w377:dbl, "Error Out"=w376:errorcluster)  [unwired: 10 in]
        n163 = call "uc480_SubVI_Example_GetPixelClock.vi"(".NET (Reference)"=w366, "Error In"=w376) -> ("Pixel Clock"=w381:i32, "Inc"=w383:i32, "Min"=w384:i32, "Max"=w385:i32, "error out"=w382:errorcluster)  [unwired: 9 in]
        n164 = property on="Pixelclock" class="Slide (strict)"(error in=w382, "Value"=w381, "Increment"=w383, "Minimum"=w384, "Maximum"=w385) -> (error out=w386:errorcluster)  [unwired: 1 in, 1 out]
        n165 = property on="Pixelclock" class="Slide (strict)"(error in=w386, "Scale.Increment"=w383, "Scale.Minimum"=w384, "Scale.Maximum"=w385) -> (error out=w387:errorcluster)  [unwired: 1 in, 1 out]
        n166 = call "uc480_SubVI_Example_GetFramerate.vi"(".NET (Reference)"=w366, "Error In"=w387) -> ("Framerate"=w390:dbl, "Inc"=w391:dbl, "Min"=w392:dbl, "Max"=w393:dbl, "error out"=w389:errorcluster)  [unwired: 9 in]
        n167 = property on="Framerate" class="Slide (strict)"(error in=w389, "Value"=w390, "Increment"=w391, "Minimum"=w392, "Maximum"=w393) -> (error out=w388:errorcluster)  [unwired: 1 in, 1 out]
        n168 = property on="Framerate" class="Slide (strict)"(error in=w388, "Scale.Increment"=w391, "Scale.Minimum"=w392, "Scale.Maximum"=w393) -> (error out=w394:errorcluster)  [unwired: 1 in, 1 out]
        n169 = call "uc480_SubVI_Example_GetExposure.vi"(".NET (Reference)"=w366, "Error In"=w394) -> ("Exposure"=w397:dbl, "Inc"=w398:dbl, "Min"=w399:dbl, "Max"=w400:dbl, "Error out"=w395:errorcluster)  [unwired: 9 in]
        n170 = property on="Exposure" class="Slide (strict)"(error in=w395, "Value"=w397, "Increment"=w398, "Minimum"=w399, "Maximum"=w400) -> (error out=w396:errorcluster)  [unwired: 1 in, 1 out]
        n171 = property on="Exposure" class="Slide (strict)"(error in=w396, "Scale.Increment"=w398, "Scale.Minimum"=w399, "Scale.Maximum"=w400) -> (error out=w375:errorcluster)  [unwired: 1 in, 1 out]
        n172 = call "uc480_SubVI_Example_Timing.vi"(".NET (Reference)"=w366, "Pixelclock"=w379, "Exposure time"=w378, "Framerate"=w377, "Error In"=w375) -> ("Error Out"=w365:errorcluster)  [unwired: 7 in, 3 out]
        n173 = call "uc480_SubVI_Example_Is_XS.vi"("Error In"=w365, ".NET (Reference)"=w366) -> ("Error Out"=w362:errorcluster, "IsXS"=w364:bool)  [unwired: 7 in, 1 out]
        n174 = case shown="False" w364 {
          tunnel: w362 -> [w431 w444]
          tunnel: [w431 w444] -> w363
          frame False {
            n175 = control-ref of="Pixelclock"() -> (w427:refnum<vi>)
            n176 = control-ref of="Framerate"() -> (w426:refnum<vi>)
            n177 = control-ref of="Exposure"() -> (w425:refnum<vi>)
            n178 = property class="Slide (strict)"(reference=w427, "DisabledEnum"=T6."Enabled" ("Disabled")) -> (reference out=w424:refnum<vi>, error out=w423:errorcluster)  [unwired: 1 in]
            n179 = property class="Slide (strict)"(reference=w426, "DisabledEnum"=T6."Enabled" ("Disabled")) -> (reference out=w422:refnum<vi>, error out=w421:errorcluster)  [unwired: 1 in]
            n180 = property class="Slide (strict)"(reference=w425, "DisabledEnum"=T6."Enabled" ("Disabled")) -> (reference out=w420:refnum<vi>, error out=w419:errorcluster)  [unwired: 1 in]
            n181 = Close Reference(reference=w424, error in (no error)=w423) -> ()  [unwired: 1 out]
            n182 = Close Reference(reference=w422, error in (no error)=w421) -> ()  [unwired: 1 out]
            n183 = Close Reference(reference=w420, error in (no error)=w419) -> ()  [unwired: 1 out]
          }
          frame True {
            n184 = control-ref of="Pixelclock"() -> (w443:refnum<vi>)
            n185 = control-ref of="Framerate"() -> (w440:refnum<vi>)
            n186 = control-ref of="Exposure"() -> (w438:refnum<vi>)
            n187 = property class="Slide (strict)"(reference=w443, "DisabledEnum"=T6."Disabled and Grayed Out" ("Disabled")) -> (reference out=w436:refnum<vi>, error out=w437:errorcluster)  [unwired: 1 in]
            n188 = property class="Slide (strict)"(reference=w440, "DisabledEnum"=T6."Disabled and Grayed Out" ("Disabled")) -> (reference out=w435:refnum<vi>, error out=w434:errorcluster)  [unwired: 1 in]
            n189 = property class="Slide (strict)"(reference=w438, "DisabledEnum"=T6."Disabled and Grayed Out" ("Disabled")) -> (reference out=w433:refnum<vi>, error out=w432:errorcluster)  [unwired: 1 in]
            n190 = Close Reference(reference=w436, error in (no error)=w437) -> ()  [unwired: 1 out]
            n191 = Close Reference(reference=w435, error in (no error)=w434) -> ()  [unwired: 1 out]
            n192 = Close Reference(reference=w433, error in (no error)=w432) -> ()  [unwired: 1 out]
          }
        }
        n193 = call "uc480_SubVI_Example_MemoryAllocation.vi"(".NET (Reference)"=w366, "Error In"=w363) -> ("Bits/Pixel 2"=→"Bits/Pixel":i32, "Width"=→"Width":i32, "Serial Number"=→"Serial Number":string, "Height"=→"Height":i32, "Error Out"=w405:errorcluster)  [unwired: 13 in]
      }
      frame "Start live" {
        # "Has acquisition started?"
        # "Start Acquisition"
        n194 = property class="Camera"(reference=w461, error in=w462) -> (error out=w471:errorcluster, "Acquisition"=w470:refnum<k24>)  [unwired: 1 out]
        n195 = invoke class="Acquisition" method="HasStarted"(reference=w470, error in=w471) -> (reference out=w466:refnum<k24>, error out=w465:errorcluster, "HasStarted"=w464:i32, "bValue"=w469:bool)  [unwired: 2 in]
        n196 = control-ref of="Load Parameter"() -> (w454:refnum<vi>)
        n197 = control-ref of="Stop Live"() -> (w452:refnum<vi>)
        n198 = control-ref of="Start Live"() -> (w457:refnum<vi>)
        n199 = property class="Bool"(reference=w452, "Disabled"=u8 0 ("Deaktiviert")) -> (reference out=w450:refnum<vi>, error out=w449:errorcluster)  [unwired: 1 in]
        n200 = property class="Bool"(reference=w457, "Disabled"=u8 2 ("Deaktiviert")) -> (reference out=w446:refnum<vi>, error out=w445:errorcluster)  [unwired: 1 in]
        n201 = property class="Bool"(reference=w454, "Disabled"=u8 2 ("Deaktiviert")) -> (reference out=w448:refnum<vi>, error out=w447:errorcluster)  [unwired: 1 in]
        n202 = invoke class="Acquisition" method="ToString"(reference=w466, error in=w465) -> (error out=w468:errorcluster, "ToString"=w467:string)  [unwired: 1 in, 1 out]
        n203 = call "uc480_Error_Handling.vi"("Error Code"=w464, "Error String"=w467, "Error In"=w468) -> ("Error Out"=w463:errorcluster)  [unwired: 8 in]
        n204 = Close Reference(reference=w450, error in (no error)=w449) -> ()  [unwired: 1 out]
        n205 = Close Reference(reference=w446, error in (no error)=w445) -> ()  [unwired: 1 out]
        n206 = Close Reference(reference=w448, error in (no error)=w447) -> ()  [unwired: 1 out]
        n207 = case shown="False" w469 {
          tunnel: [w474 w484] -> w458
          tunnel: w463 -> [w480 w484]
          tunnel: w461 -> [w479 w483]
          tunnel: [w479 w483] -> w460
          frame False {
            w472 = 1 items=["IS_DONT_WAIT", "IS_WAIT"] ("Wait")
            n208 = property class="Camera"(reference=w479, error in=w480) -> (error out=w481:errorcluster, "Acquisition"=w482:refnum<k24>)  [unwired: 1 out]
            n209 = invoke class="Acquisition" method="Capture"(reference=w482, error in=w481, "param"=w472) -> (reference out=w475:refnum<k24>, error out=w476:errorcluster, "Capture"=w473:i32)  [unwired: 1 in, 1 out]
            n210 = invoke class="Acquisition" method="ToString"(reference=w475, error in=w476) -> (error out=w478:errorcluster, "ToString"=w477:string)  [unwired: 1 in, 1 out]
            n211 = call "uc480_Error_Handling.vi"("Error Code"=w473, "Error String"=w477, "Error In"=w478) -> ("Error Out"=w474:errorcluster)  [unwired: 8 in]
          }
          frame True {
          }
        }
      }
    }
    n212 = call "uc480_SubVI_Example_SyncEventLoop.vi"("Error In"=w77, "use sync"=w79, ".NET (Reference)"=w78) -> ("Error Out"=w75:errorcluster, "Synchronize (ms)"=w76:dbl)  [unwired: 7 in]
    "Error Out" <- w75
    n213 = Wait Until Next ms Multiple(millisecond multiple=w76) -> ()  [unwired: 1 out]
  }
  n214 = property class="KCubeInertialMotorControl"(reference=w67) -> (reference out=w66:refnum<k24>, "Device"=w43:refnum<k24>)  [unwired: 1 in, 1 out]
  n215 = property class="KCubeDCServoControl"(reference=w64) -> (reference out=w51:refnum<k24>, error out=w48:errorcluster, "Device"=w49:refnum<k24>)  [unwired: 1 in]
  n216 = property class="KCubeDCServoControl"(reference=w57) -> (reference out=w47:refnum<k24>, error out=w45:errorcluster, "Device"=w44:refnum<k24>)  [unwired: 1 in]
  n217 = call <vilib>:"Initialize Joystick.vi"() -> ("error out"=w52:errorcluster, "device ID"=w53:refnum<k1>)  [unwired: 10 in]
  n218 = call <vilib>:"Initialize Mouse.vi"() -> ("error out"=w5:errorcluster, "device ID"=w6:refnum<k1>)  [unwired: 10 in]
  n219 = while {
    tunnel: w66 -> [w642]
    tunnel: [w642] -> w65
    tunnel: w43 -> [w600]
    tunnel: [w632] -> w55
    tunnel: [w633] -> w54
    tunnel: w53 -> [w636]
    tunnel: w52 -> [w635]
    tunnel: w51 -> [w631]
    tunnel: [w631] -> w50
    tunnel: w49 -> [w529]
    tunnel: [w630] -> w37
    tunnel: w48 -> [w528]
    tunnel: [w625] -> w40
    tunnel: [w624] -> w46
    tunnel: w47 -> [w624]
    tunnel: w45 -> [w530]
    tunnel: w44 -> [w531]
    tunnel: [w605] -> w39
    tunnel: [w606] -> w38
    tunnel: [w591] -> w41
    tunnel: [w568] -> w42
    tunnel: [w561] -> w36
    shift-right: [w535] -> _
    shift-left: _ -> [w506]
    shift-right: [w533] -> _
    shift-left: _ -> [w501]
    shift-right: [w532] -> _
    shift-left: _ -> [w494]
    shift-right: [w534] -> _
    shift-left: _ -> [w503]
    tunnel: w6 -> [w539]
    tunnel: w5 -> [w538]
    tunnel: [w537] -> w4
    tunnel: [w536] -> w3
    tunnel: [w526] -> w2
    tunnel: [w525] -> w1
    stop <- w634 stop-if-true
    w588 = 1 items=["Channel1"=1, "Channel2"=2, "Channel3"=3, "Channel4"=4] ("channel")
    w601 = 1 items=["Channel1"=1, "Channel2"=2, "Channel3"=3, "Channel4"=4] ("channel 2")
    (unwired) 1 items=["Channel1"=1, "Channel2"=2, "Channel3"=3, "Channel4"=4] ("channel")
    n220 = call-poly <vilib>:"Acquire Input Data.vi"("device ID"=w636, "error in (no error)"=w635) -> ("device ID"=w633:refnum<k1>, "axis info"=w638:T4, "button info"=w629:T5, "direction info"=w621:T3, "error out"=w632:errorcluster)  [unwired: 13 in]
    "axis info 2" <- w638
    "direction info 2" <- w621
    "button info 2" <- w629
    n221 = call-poly <vilib>:"Acquire Input Data.vi"("device ID"=w539, "error in (no error)"=w538) -> ("device ID"=w537:refnum<k1>, "axis info"=w549:T7, "button info"=w547:T8, "error out"=w536:errorcluster)  [unwired: 14 in]
    n222 = Wait (ms)(milliseconds to wait=u32 50) -> ()  [unwired: 1 out]
    n223 = Unbundle(w621) -> ()  [unwired: 4 out]
    n224 = Unbundle(w621) -> ()  [unwired: 4 out]
    n225 = Unbundle(w621) -> ()  [unwired: 4 out]
    n226 = Unbundle By Name(w547) -> ("button 1"=w486:bool, "button 2"=w546:bool)
    "button 1" <- w486
    "button 2" <- w546
    n227 = Unbundle(w549) -> ("Horizontal"=w545:i32, "Vertical"=w542:i32, "Scrolling"=→"Scrolling":i32)
    n228 = Unbundle By Name(w638) -> ("X axis"=w639:i32, "Z axis"=w615:i32, "Z axis rotation"=w581:i32)  [unwired: 5 out]
    n229 = call "Elapsed Time"() -> ("Elapsed Time (s)"=→"Time the program is running (s)":dbl)  [unwired: 12 in, 7 out]
    n230 = Or(x=w632, y="?") -> (x .or. y?=w634:bool)
    n231 = Unbundle(w629) -> ("button 1"=w555:bool, "button 2"=w557:bool, "button 3"=w554:bool, "button 4"=w556:bool, "button 7"=→"Moving":bool, "button 8"=w570:bool)  [unwired: 26 out]
    "You are Sprinting now" <- w570
    n232 = case shown="True" w555 {
      tunnel: [w753 w759] -> w626
      tunnel: w529 -> [w753 w756]
      tunnel: [w752 w755] -> w627
      tunnel: w528 -> [w752 w754]
      frame False {
      }
      frame True {
        w758 = 2 items=["Forward"=1, "Backward"=2] ("direction")
        n233 = invoke class="KCubeDCServo" method="MoveJog"(reference=w756, error in=w754, "direction"=w758, "waitTimeout"=0) -> (reference out=w759:refnum<k24>, error out=w755:errorcluster)  [unwired: 1 in, 3 out]
      }
    }
    n234 = case shown="True" w554 {
      tunnel: w529 -> [w760 w765]
      tunnel: [w761 w764] -> w628
      tunnel: w528 -> [w761 w763]
      tunnel: [w760 w762] -> w596
      frame False {
      }
      frame True {
        w767 = 1 items=["Forward"=1, "Backward"=2] ("direction")
        n235 = invoke class="KCubeDCServo" method="MoveJog"(reference=w765, error in=w763, "direction"=w767, "waitTimeout"=5000) -> (reference out=w762:refnum<k24>, error out=w764:errorcluster)  [unwired: 1 in, 3 out]
      }
    }
    n236 = case shown="True" w557 {
      tunnel: [w672 w678] -> _
      tunnel: w531 -> [w672 w675]
      tunnel: [w671 w674] -> w568
      tunnel: w530 -> [w671 w673]
      frame False {
      }
      frame True {
        w677 = 2 items=["Forward"=1, "Backward"=2] ("direction")
        n237 = invoke class="KCubeDCServo" method="MoveJog"(reference=w675, error in=w673, "direction"=w677, "waitTimeout"=0) -> (reference out=w678:refnum<k24>, error out=w674:errorcluster)  [unwired: 1 in, 3 out]
      }
    }
    n238 = case shown="True" w556 {
      tunnel: w531 -> [w679 w684]
      tunnel: [w680 w683] -> w566
      tunnel: w530 -> [w680 w682]
      tunnel: [w679 w681] -> w582
      frame False {
      }
      frame True {
        w686 = 1 items=["Forward"=1, "Backward"=2] ("direction")
        n239 = invoke class="KCubeDCServo" method="MoveJog"(reference=w684, error in=w682, "direction"=w686, "waitTimeout"=5000) -> (reference out=w681:refnum<k24>, error out=w683:errorcluster)  [unwired: 1 in, 3 out]
      }
    }
    n240 = Multiply(x=w639, y=1) -> (x*y=w640:i32)
    n241 = Add(x=w581, y=256) -> (x+y=w559:i32)
    n242 = Subtract(x=w545, y=0) -> (x-y=w543:i32)
    "Horizontal" <- w543
    n243 = Subtract(x=w542, y=0) -> (x-y=w541:i32)
    "Vertical" <- w541
    n244 = Select(t=3430.4, s=w570, f=343.04) -> (s? t:f=w610:dbl)
    n245 = Select(t=3430.4, s=w570, f=343.04) -> (s? t:f=w574:dbl)
    n246 = Multiply(x=-1, y=w559) -> (x*y=w560:i32)
    n247 = Divide(x=w640, y=1000) -> (x/y=w595:dbl)
    n248 = Multiply(x=w610, y=w615) -> (x*y=w619:dbl)
    n249 = Multiply(x=w574, y=w560) -> (x*y=w578:dbl)
    n250 = case shown="True" w486 {
      tunnel: w543 -> [_ w658]
      tunnel: w541 -> [_ w657]
      tunnel: [w656 w658] -> w533
      tunnel: [w655 w657] -> w532
      tunnel: w501 -> [w656 _]
      tunnel: w494 -> [w655 _]
      frame False {
      }
      frame True {
      }
    }
    n251 = case shown="True" w546 {
      tunnel: [w660 w662] -> w534
      tunnel: w543 -> [_ w662]
      tunnel: [w659 w661] -> w535
      tunnel: w541 -> [_ w661]
      tunnel: w503 -> [w660 _]
      tunnel: w506 -> [w659 _]
      frame False {
      }
      frame True {
      }
    }
    n252 = Divide(x=w619, y=327670.0) -> (x/y=w598:dbl)
    n253 = Divide(x=w578, y=327670.0) -> (x/y=w572:dbl)
    n254 = Divide(x=w598, y=5.0) -> (x/y=w597:dbl)
    n255 = Equal?(x=w560, y=0.0) -> (x = y?=w562:bool)
    n256 = Divide(x=w572, y=5.0) -> (x/y=w571:dbl)
    n257 = invoke class="KCubeDCServo" method="GetPositionCounter"(reference=w626, error in=w627) -> (error out=w625:errorcluster)  [unwired: 1 in, 2 out]
    n258 = invoke class="KCubeDCServo" method="GetPositionCounter"(reference=w596, error in=w628) -> (reference out=w616:refnum<k24>, error out=w630:errorcluster, "GetPositionCounter"=w584:i32)  [unwired: 1 in]
    n259 = invoke class="KCubeDCServo" method="GetPositionCounter"(reference=w582, error in=w566) -> (reference out=w567:refnum<k24>, "GetPositionCounter"=w569:i32)  [unwired: 1 in, 1 out]
    n260 = Subtract(x=w506, y="a") -> (x-y=w493:dbl)
    "upper verti limit" <- w493
    n261 = Subtract(x=w503, y=w501) -> (x-y=w524:i32)
    n262 = Add(x=w584, y=w597) -> (x+y=w553:dbl)
    n263 = Add(x=w569, y=w571) -> (x+y=w565:dbl)
    n264 = Equal?(x=w615, y=0.0) -> (x = y?=w617:bool)
    n265 = Multiply(x=w524, y=34304) -> (x*y=w522:i32)
    n266 = case shown="False" w617 {
      tunnel: w616 -> [w746 w750]
      tunnel: w528 -> [w747 w751]
      tunnel: [w749 w751] -> w614
      tunnel: [w745 w750] -> w613
      tunnel: w553 -> [w744 _]
      frame False {
        n267 = invoke class="KCubeDCServo" method="MoveTo_DeviceUnit"(reference=w746, error in=w747, "position"=w744, "waitTimeout"=0) -> (reference out=w745:refnum<k24>, error out=w749:errorcluster)  [unwired: 1 in, 3 out]
      }
      frame True {
      }
    }
    n268 = case shown="False" w562 {
      tunnel: w567 -> [w667 w669]
      tunnel: w566 -> [w666 w670]
      tunnel: w565 -> [w665 _]
      tunnel: [w664 w669] -> w564
      tunnel: [w663 w670] -> w563
      frame False {
        n269 = invoke class="KCubeDCServo" method="MoveTo_DeviceUnit"(reference=w667, error in=w666, "position"=w665, "waitTimeout"=0) -> (reference out=w664:refnum<k24>, error out=w663:errorcluster)  [unwired: 1 in, 3 out]
      }
      frame True {
      }
    }
    n270 = Divide(x=w522, y="1mm=?pixel") -> (x/y=w509:dbl)
    "Numeric2" <- w509
    n271 = Subtract(x=w506, y=w494) -> (x-y=w521:i32)
    n272 = Multiply(x=w521, y=34304) -> (x*y=w519:i32)
    n273 = Divide(x=w519, y="1mm=?pixel") -> (x/y=w508:dbl)
    "Numeric1" <- w508
    n274 = Add(x=w506, y="b") -> (x+y=w492:dbl)
    "lower verti limit" <- w492
    n275 = invoke class="KCubeDCServo" method="GetPositionCounter"(reference=w613, error in=w614) -> (reference out=w608:refnum<k24>, error out=w605:errorcluster, "GetPositionCounter"=w517:i32)  [unwired: 1 in]
    n276 = Add(x=w517, y=w509) -> (x+y=w515:dbl)
    n277 = Divide(x=w515, y=34304.0) -> (x/y=→"motor 2":dbl)
    n278 = invoke class="KCubeDCServo" method="GetPositionCounter"(reference=w564, error in=w563) -> (error out=w561:errorcluster, "GetPositionCounter"=w516:i32)  [unwired: 1 in, 1 out]
    n279 = Add(x=w516, y=w508) -> (x+y=w511:dbl)
    n280 = Divide(x=w511, y=34304.0) -> (x/y=→"motor 1":dbl)
    n281 = Divide(x=w517, y=34304.0) -> (x/y=w607:dbl)
    "position of motor 1 (mm)" <- w607
    n282 = Divide(x=w516, y=34304) -> (x/y=→"position of motor 2 (mm)":dbl)
    n283 = Subtract(x=w503, y="c") -> (x-y=w500:dbl)
    "left hori limit" <- w500
    n284 = Add(x=w503, y="d") -> (x+y=w499:dbl)
    "right hori limit" <- w499
    n285 = case shown="True" "Move motor control" {
      tunnel: w608 -> [_ w696]
      tunnel: w607 -> [_ w695]
      tunnel: [w687 w694] -> w606
      tunnel: w605 -> [w687 w693]
      tunnel: w517 -> [_ w692]
      tunnel: "end pos (mm)" -> [_ w691]
      tunnel: "step size (mm) 2" -> [_ w690]
      tunnel: "Cancel Button" -> [_ w689]
      tunnel: "Cancel Button" -> [_ w688]
      frame False {
      }
      frame True {
        n286 = Greater Or Equal?(x=w695, y=w691) -> (x >= y?=w697:bool)
        n287 = case shown="True" w697 {
          tunnel: w696 -> [w704 w727]
          tunnel: w691 -> [w703 w726]
          tunnel: [w702 w725] -> w694
          tunnel: w693 -> [w701 w724]
          tunnel: w692 -> [w700 w723]
          tunnel: w690 -> [w699 w722]
          tunnel: w689 -> [_ w721]
          tunnel: w688 -> [w698 _]
          frame False {
            n288 = while {
              tunnel: w704 -> [w717]
              tunnel: [w720] -> _
              tunnel: w703 -> [w720]
              tunnel: [w715] -> w702
              tunnel: w701 -> [w716]
              tunnel: w700 -> [w710]
              tunnel: w699 -> [w711]
              tunnel: w698 -> [w708]
              stop <- w705 stop-if-true
              n289 = Wait (ms)(milliseconds to wait=u32 50) -> ()  [unwired: 1 out]
              n290 = Multiply(x=w711, y=34304.0) -> (x*y=w712:dbl)
              n291 = Add(x=w710, y=w712) -> (x+y=w714:dbl)
              n292 = invoke class="KCubeDCServo" method="MoveTo_DeviceUnit"(reference=w717, error in=w716, "position"=w714, "waitTimeout"=0) -> (error out=w715:errorcluster)  [unwired: 1 in, 4 out]
              n293 = Greater Or Equal?(x=w714, y=w720) -> (x >= y?=w709:bool)
              n294 = Or(x=w708, y=w709) -> (x .or. y?=w706:bool)
              n295 = Or(x="stop", y=w706) -> (x .or. y?=w705:bool)
            }
          }
          frame True {
            n296 = while {
              tunnel: w727 -> [w738]
              tunnel: [w739] -> _
              tunnel: w726 -> [w739]
              tunnel: [w737] -> w725
              tunnel: w724 -> [w740]
              tunnel: w723 -> [w733]
              tunnel: w722 -> [w734]
              tunnel: w721 -> [w731]
              stop <- w728 stop-if-true
              n297 = Wait (ms)(milliseconds to wait=u32 50) -> ()  [unwired: 1 out]
              n298 = Multiply(x=w734, y=-34300.0) -> (x*y=w735:dbl)
              n299 = Add(x=w733, y=w735) -> (x+y=w741:dbl)
              n300 = invoke class="KCubeDCServo" method="MoveTo_DeviceUnit"(reference=w738, error in=w740, "position"=w741, "waitTimeout"=0) -> (error out=w737:errorcluster)  [unwired: 1 in, 4 out]
              n301 = Less?(x=w741, y=w739) -> (x < y?=w732:bool)
              n302 = Or(x=w731, y=w732) -> (x .or. y?=w729:bool)
              n303 = Or(x="stop 2", y=w729) -> (x .or. y?=w728:bool)
            }
          }
        }
      }
    }
    n304 = Less Or Equal?(x=w501, y=w499) -> (x <= y?=w498:bool)
    n305 = Greater Or Equal?(x=w501, y=w500) -> (x >= y?=w497:bool)
    n306 = And(x=w498, y=w497) -> (x .and. y?=w491:bool)
    n307 = Greater Or Equal?(x=w494, y=w493) -> (x >= y?=w495:bool)
    n308 = Less Or Equal?(x=w494, y=w492) -> (x <= y?=w496:bool)
    n309 = And(x=w496, y=w495) -> (x .and. y?=w490:bool)
    n310 = invoke on="Invoke Node" class="KCubeInertialMotor" method="GetPosition"(reference=w600, "channel"=w601) -> (reference out=w587:refnum<k24>, error out=w586:errorcluster, "GetPosition"=w585:i32)  [unwired: 2 in, 1 out]
    "Position of z direction" <- w585
    n311 = And(x=w490, y=w491) -> (x .and. y?=w489:bool)
    n312 = Add(x=w585, y=w595) -> (x+y=w590:dbl)
    n313 = invoke class="KCubeInertialMotor" method="MoveTo"(reference=w587, error in=w586, "channel"=w588, "position"=w590, "waitTimeout"=0) -> (reference out=w593:refnum<k24>, error out=w592:errorcluster)  [unwired: 1 in, 4 out]
    n314 = And(x=w489, y="ready to use mouse?") -> (x .and. y?=w487:bool)
    "in screen?" <- w487
    n315 = invoke on="Invoke Node" class="KCubeInertialMotor" method="GetPosition"(reference=w593, error in=w592, "channel"="channel 3") -> (error out=w591:errorcluster)  [unwired: 1 in, 3 out]
    n316 = And(x=w487, y=w486) -> (x .and. y?=w485:bool)
    "blinker and move" <- w485
    n317 = case shown="True" w485 {
      tunnel: w531 -> [_ w654]
      tunnel: w530 -> [w644 w653]
      tunnel: w529 -> [_ w652]
      tunnel: w528 -> [w643 w651]
      tunnel: w517 -> [_ _]
      tunnel: [w643 w648] -> w526
      tunnel: [w644 w647] -> w525
      tunnel: w515 -> [_ w646]
      tunnel: w511 -> [_ w645]
      frame False {
      }
      frame True {
        n318 = invoke class="KCubeDCServo" method="MoveTo_DeviceUnit"(reference=w654, error in=w653, "position"=w646, "waitTimeout"=0) -> (error out=w647:errorcluster)  [unwired: 1 in, 4 out]
        n319 = invoke class="KCubeDCServo" method="MoveTo_DeviceUnit"(reference=w652, error in=w651, "position"=w645, "waitTimeout"=0) -> (error out=w648:errorcluster)  [unwired: 1 in, 4 out]
      }
    }
    "Horizontal right click" <- w503
    "Vertical right click" <- w506
    "Horizontal left click" <- w501
    "Vertical left click" <- w494
    "Move motor indicator" <- "Move motor control"
  }
  "error out 5" <- w42
  "error out" <- w41
  "error out 2" <- w40
  "error out 3" <- w39
  "error out 4" <- w38
  "error out 6" <- w37
  "error out 7" <- w36
  "error out 8" <- w2
  "error out 9" <- w1
  n320 = invoke class="KCubeInertialMotorControl" method="CloseDevice"(reference=w65) -> ()  [unwired: 2 in, 3 out]
  n321 = invoke class="KCubeDCServoControl" method="CloseDevice"(reference=w50) -> ()  [unwired: 2 in, 3 out]
  n322 = invoke class="KCubeDCServoControl" method="CloseDevice"(reference=w46) -> ()  [unwired: 2 in, 3 out]
  n323 = call-poly <vilib>:"Close Input Device.vi"("error in (no error)"=w3, "device ID"=w4) -> ()  [unwired: 8 in, 1 out]
  n324 = call-poly <vilib>:"Close Input Device.vi"("error in (no error)"=w55, "device ID"=w54) -> ("error out"=w56:errorcluster)  [unwired: 8 in]
  n325 = call <vilib>:"Simple Error Handler.vi"("error in (no error)"=w56) -> ()  [unwired: 4 in, 5 out]
